vi "Create Stiffness Records.vi"(1 "Step":string, 3 "Stiffness Updates":T2[](array[typedef]), 4 "Timestamp":timestamp) -> (0 "Records":string[](array[string]))   [LabVIEW 2009]
uses:
  Global Data/Jacobian Stiffness Column.ctl
  Global Data/Jacobian Stiffness Column Id.ctl
  Archive File Type.ctl
panel:
  in  "Active Matrices":T1[](array[typedef])
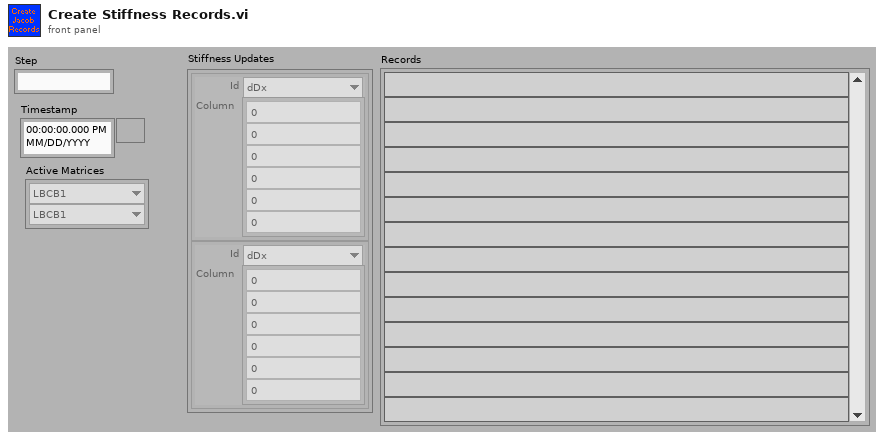
[diagram p1: front panel]
types:
  T1 = typedef "Archive File Type.ctl" = enum16{"LBCB1", "LBCB2", "ExternalSensors", "Combined"}
  T2 = typedef "Jacobian Stiffness Column.ctl" = cluster{"Id":T3, "Column":dbl[]}
  T3 = typedef "Jacobian Stiffness Column Id.ctl" = enum16{"dDx", "dDy", "dDz", "dRx", "dRy", "dRz"}
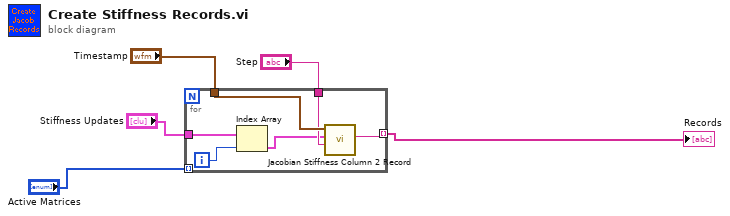
[diagram p0: block diagram]
diagram:
  n1 = for {
    tunnel: "Timestamp" -> [w11]
    tunnel: [w10] -> w1 mode=indexing
    tunnel: "Step" -> [w9]
    tunnel: "Active Matrices" -> [_] mode=indexing
    tunnel: "Stiffness Updates" -> [w7]
    i -> [w6]
    n2 = Index Array(array=w7, index=w6) -> (element=w8:T2)
    n3 = call "Jacobian Stiffness Column 2 Record.vi"("Step"=w9, "Jacobian Stiffness Column"=w8, "Time Stamp"=w11) -> ("Record"=w10:string)  [unwired: 8 in]
  }
  "Records" <- w1
